vi "read_params.vi"(8 "error in (no error)":errorcluster, 11 "RidgeClassifier in":refnum<class "RidgeClassifier.lvclass">) -> (0 "error out":errorcluster, 2 "params":T1={"alpha"=1.0, "fit_intercept"=TRUE, "normalize"=FALSE, "copy_X"=TRUE, "max_iter"={"max_iter_type"="None", "max_iter_int"=0.0}, "tol"=0.001, "class_weight"={"class_weight_type"="None", "class_weight_dict"="{0:1.2,1:0.8,2:1.0}"}, "solver"="auto", "random_state"=0.0}, 3 "RidgeClassifier out":refnum<class "RidgeClassifier.lvclass">)   [LabVIEW 2020, in "RidgeClassifier.lvclass"]
uses:
  RidgeClassifier.lvclass
  Controls/ridge_classifier_params.ctl
  RidgeClassifier.lvclass/RidgeClassifier.ctl
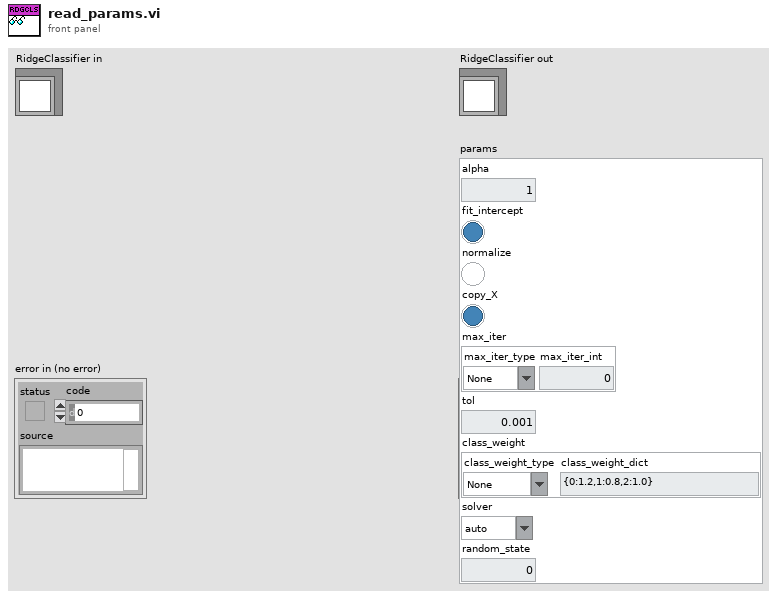
[diagram p1: front panel]
types:
  T1 = typedef "ridge_classifier_params.ctl" = cluster{"alpha":dbl, "fit_intercept":bool, "normalize":bool, "copy_X":bool, "max_iter":cluster{"max_iter_type":string, "max_iter_int":dbl}, "tol":dbl, "class_weight":cluster{"class_weight_type":string, "class_weight_dict":string}, "solver":string, "random_state":dbl}
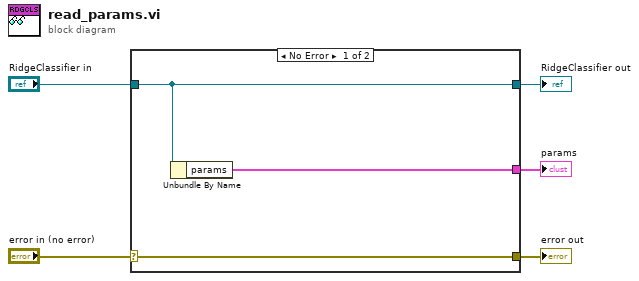
[diagram p0: block diagram]
diagram:
  n1 = case shown="No Error" "error in (no error)" {
    selector: "error in (no error)" -> [w8 w9]
    tunnel: [w8 w9] -> w4
    tunnel: [w7 w10] -> w2
    tunnel: "RidgeClassifier in" -> [w7 w10]
    tunnel: [w6 _] -> w1
    frame No Error {
      n2 = Unbundle By Name(w7) -> ("params"=w6:T1)
    }
    frame Error {
    }
  }
  "error out" <- w4
  "RidgeClassifier out" <- w2
  "params" <- w1
